vi "Send value.vi"(3 "Error In":errorcluster, 4 "Output (0...1)":sgl, 5 "Port":refnum<visa-resource-name>) -> (0 "Error Out":errorcluster, 1 "Output":sgl, 2 "Port out":refnum<visa-resource-name>)   [LabVIEW 2016]
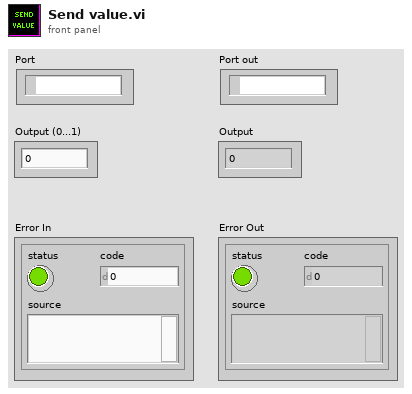
[diagram p1: front panel]
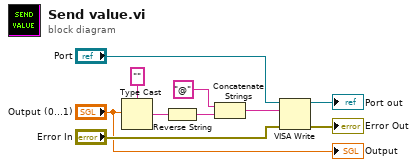
[diagram p0: block diagram]
diagram:
  n1 = Type Cast(type="", x="Output (0...1)") -> (*(type *) &x=w9:string)
  n2 = Reverse String(1:w9) -> (0:w8:string)
  n3 = Concatenate Strings("@", w8) -> (w6:string)
  n4 = VISA Write(VISA resource name="Port", write buffer=w6, error in (no error)="Error In") -> (VISA resource name out=→"Port out":refnum<visa-resource-name>, error out=→"Error Out":errorcluster)  [unwired: 1 out]
  "Output" <- "Output (0...1)"
